vi "Update Status.vi"(8 "error in (no error)":errorcluster, 11 "Framework in":refnum<class "Framework.lvclass">) -> (0 "error out":errorcluster, 3 "Framework out":refnum<class "Framework.lvclass">)   [LabVIEW 2017, in "DSF Core.lvlib" / "Framework.lvclass"]
uses:
  Framework.lvclass
  Framework.lvclass/Framework.ctl
  Framework Status/Framework Status.lvclass/Framework Status.ctl
  Status/Status Data.ctl
  <vilib>/NI/Memory Manager/Classes/Pointer/Pointer.lvclass/Pointer.ctl
  Plugin/Plugin.lvclass/Plugin.ctl
  Timing/Timing.lvclass/Timing.ctl
  <vilib>/NI/Memory Manager/Classes/Pointer/Get Address.vi
  Transfer Group Status/Status Size.vi
  <vilib>/NI/Memory Manager/Classes/Pointer/Check Null Pointer.vi
  <vilib>/NI/Memory Manager/Classes/Pointer/Check Size (0D).vi
  Timing/Get Iteration.vi
  <vilib>/NI/Memory Manager/Classes/Pointer/Errors.vi
  <vilib>/NI/Memory Manager/Classes/Pointer/Null Pointer.vi
  <vilib>/NI/Memory Manager/Classes/Pointer/Is Null.vi
  <vilib>/NI/Memory Manager/Classes/Pointer/Out of Bounds.vi
  <vilib>/NI/Memory Manager/Classes/Pointer/Get Size.vi
  <vilib>/NI/Memory Manager/Classes/Pointer/Create Error.vi
  <vilib>/NI/Memory Manager/VIs/Source.Write.String.vi
  <vilib>/NI/Memory Manager/Classes/Pointer/Write Pointer Size.vi
  <vilib>/NI/Memory Manager/VIs/Source.Write.Scalar.Base10.vi
  <vilib>/NI/Memory Manager/VIs/Source.Write.Scalar.Base10 (U64).vi
  <vilib>/NI/Memory Manager/VIs/New Error Cluster Constant.vi
  <vilib>/NI/Memory Manager/VIs/New Error Cluster Constant (512B).vi
  <vilib>/NI/Memory Manager/VIs/Error Cluster.Set Status.vi
  <vilib>/NI/Memory Manager/VIs/Error Cluster.Set Code.vi
  <vilib>/NI/Memory Manager/VIs/Error Cluster.Set VI Source.vi
  <vilib>/NI/Memory Manager/Constants/Constants.vi
  <vilib>/NI/Memory Manager/Constants/Library Name.vi
  <vilib>/NI/Memory Manager/Classes/Pointer/Pointer Error Info.vi
  <vilib>/NI/Memory Manager/Constants/Pointer Class Name.vi
  Transfer Group Status/Status.lvclass
  C:/Program Files (x86)/National Instruments/LabVIEW 2017/vi.lib/NI/Memory Manager/Classes/Pointer/Pointer.lvclass
  Framework Status/Framework Status.lvclass
  Plugin/Plugin.lvclass
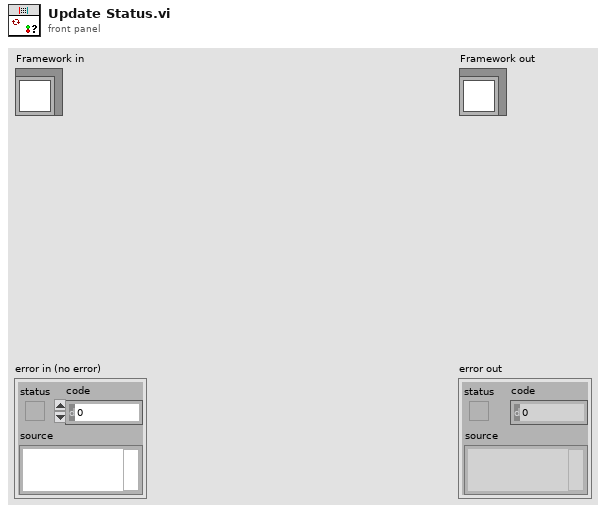
[diagram p1: front panel]
types:
  T1 = typedef "DSF Core.lvlib/Status.lvclass/Status Data.ctl" = cluster{"late count":u64, "iteration":u64, "duration":u32}
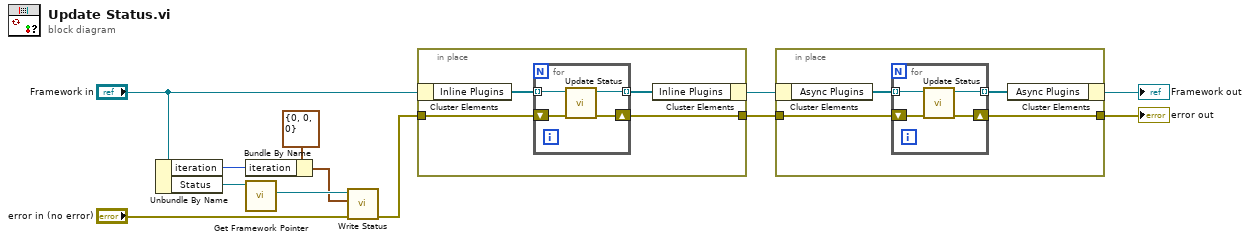
[diagram p0: block diagram]
diagram:
  n1 = Unbundle By Name("Framework in") -> ("iteration"=w8:u64, "Status"=w7:refnum<class "Framework Status.lvclass">)
  n2 = Bundle By Name(cluster=T1 {"late count"=0, "iteration"=0, "duration"=0} ("status"), "iteration"=w8) -> (w9:T1)
  n3 = call "Get Framework Pointer.vi"("Framework Status in"=w7) -> ("framework pointer"=w11:refnum<class "Status.lvclass">)  [unwired: 9 in, 1 out]
  n4 = call "Write Status.vi"("error in (no error)"="error in (no error)", "status"=w9, "status pointer in"=w11) -> ("error out"=w5:errorcluster)  [unwired: 7 in, 1 out]
  n5 = in-place {
    in-place-border: [w14] -> w3
    in-place-border: w5 -> [w13]
    n6 = in-place-cluster #1("Framework in") -> ("Inline Plugins"=w16:refnum<class "Plugin.lvclass">[])
    n7 = for {
      tunnel: w16 -> [w20] mode=indexing
      tunnel: [w19] -> w15 mode=indexing
      shift-right: [w18] -> w14
      shift-left: w13 -> [w17]
      n8 = call "Update Status.vi"("error in (no error)"=w17, "Plugin in"=w20) -> ("error out"=w18:errorcluster, "Plugin out"=w19:refnum<class "Plugin.lvclass">)  [unwired: 8 in]
    }
    n9 = in-place-cluster #1("Inline Plugins"=w15) -> (w4:refnum<class "Framework.lvclass">)
  }
  n10 = in-place {
    in-place-border: [w22] -> w1
    in-place-border: w3 -> [w21]
    n11 = in-place-cluster #2(w4) -> ("Async Plugins"=w24:refnum<class "Plugin.lvclass">[])
    n12 = for {
      tunnel: w24 -> [w28] mode=indexing
      tunnel: [w27] -> w23 mode=indexing
      shift-right: [w26] -> w22
      shift-left: w21 -> [w25]
      n13 = call "Update Status.vi"("error in (no error)"=w25, "Plugin in"=w28) -> ("error out"=w26:errorcluster, "Plugin out"=w27:refnum<class "Plugin.lvclass">)  [unwired: 8 in]
    }
    n14 = in-place-cluster #2("Async Plugins"=w23) -> (→"Framework out":refnum<class "Framework.lvclass">)
  }
  "error out" <- w1
